vi "Initialize Use Default Limits.vi"(8 "error in (no error)":errorcluster, 11 "Numeric Data Type in":refnum<class "Numeric Data Type.lvclass">) -> (0 "error out":errorcluster, 3 "Numeric Data Type (dup)":refnum<class "Numeric Data Type.lvclass">)   [LabVIEW 2018, in "Numeric Data Type.lvclass"]
uses:
  Numeric Data Type.lvclass
  Numeric Data Type.lvclass/Numeric Data Type.ctl
  Reference Use Default Limits.vi
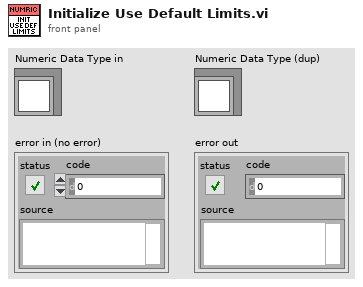
[diagram p1: front panel]
types:
  T1 = enum8{"Enabled", "Disabled", "Disabled and Grayed Out"}
  T2 = typedef "Numeric Data Type.lvclass/Representation Enum.ctl" = enum16{"Extended (EXT)", "Double (DBL)", "Single (SGL)", "Fixed-Point (FXP)", "Quad Integer (I64)", "Long Integer (I32)", "Word Integer (I16)", "Byte Integer (I8)", "Unsigned Quad (U64)", "Unsigned Long (U32)", "Unsigned Word (U16)", "Unsigned Byte (U8)", "Complex Extended (CXT)", "Complex Double (CDB)", "Complex Single (CSG)"}
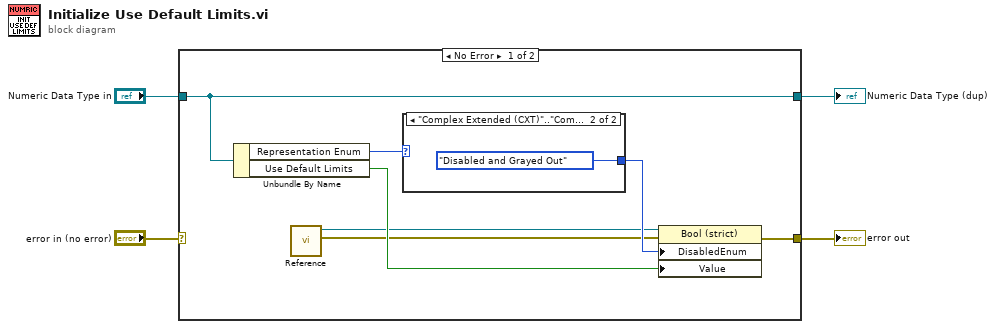
[diagram p0: block diagram]
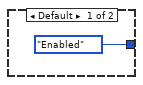
[diagram p2: hidden frame]
diagram:
  n1 = case shown="No Error" "error in (no error)" {
    selector: "error in (no error)" -> [_ w14]
    tunnel: [w8 w14] -> w4
    tunnel: "Numeric Data Type in" -> [w5 w15]
    tunnel: [w5 w15] -> w1
    frame No Error {
      n2 = Unbundle By Name(w5) -> ("Representation Enum"=w9:T2, "Use Default Limits"=w11:bool)
      n3 = call-poly "Reference.vi"() -> ("error out"=w7:errorcluster, "Use Default Limits"=w6:refnum<vi>)  [unwired: 10 in]
      n4 = case shown="\"Complex Extended (CXT)\"..\"Complex Single (CSG)\"" w9 {
        tunnel: [T1."Enabled" ("Disabled") T1."Disabled and Grayed Out" ("Disabled")] -> w10
        frame Default {
        }
        frame "Complex Extended (CXT)".."Complex Single (CSG)" {
        }
      }
      n5 = property class="Bool (strict)"(reference=w6, error in=w7, "DisabledEnum"=w10, "Value"=w11) -> (error out=w8:errorcluster)  [unwired: 1 out]
    }
    frame Error {
    }
  }
  "Numeric Data Type (dup)" <- w1
  "error out" <- w4
